vi "Share data.vi"(8 "error in (no error)":errorcluster) -> (0 "error out":errorcluster)   [LabVIEW 2015]
uses:
  shared data (name value unit).ctl
  available share data.ctl
  selected shared data.ctl
  share data command.ctl
panel:
  out "Array 3":i32[](array[numeric])
  out "Array 2":i32[](array[numeric])
  out "Array":dbl[](array[numeric])
  out "Selected Shared Data":T1
  out "Cumulative shared data sizes":i32[](array[numeric])
  out "Selected elements":i32[](array[numeric])
  in  "Tab Control":T2(tab)
  out "My data to share":T3 {"scaled" format="%.2f"}
  in  "Write":bool[](array[boolean])
  in  "My data scrollbar":i32(c297)
  in  "List of available data":i32[](listbox)
  out "Available shared data":T4 {"Shared Data"."scaled" format="%.2f"}
  in  "Data update interval (s)":sgl=5.0 min=5 max=1000 step=5
  in  "Shared Folder":path
  in  "OK":bool
  # "The share data feature enables sharing of sensor, meter, and calculated values between workstations in a laboratory. Data acquired by this instance of ProCoDA can be shared with other ProCoDA applications and shared data from other ProCoDA applications can be accessed here.\n\nSelect a shared folder that can be accessed by all ProCoDA applications that will be sharing data.\nSet the Data update interval based on the rate at which data changes. This controls both the rate at which data is written to file and read from file.\n\nOnce data sharing is configured and initiated by a data source, then it will be visible in the \"Shared data from other instances of ProCoDA\" tab.\n\nAll available data from this computer (sensors and variables) is compiled in an array and the values that are shared are based on the selected indices in the \"My data to share\" tab. Thus if the available data is modified it will shift the array and the shared variable will change. Thus it is recommended that sharing of values be used cautiously if the ProCoDA method is still being edited.\n\nShared data is read from the files based on the name of the variable. If the name of the variable is changed by the data source, then reselect the variable using this dialog box. \n\nSelect the shared data to read by highlighting the row. Multiple rows can be selected by holding the control button down while clicking."
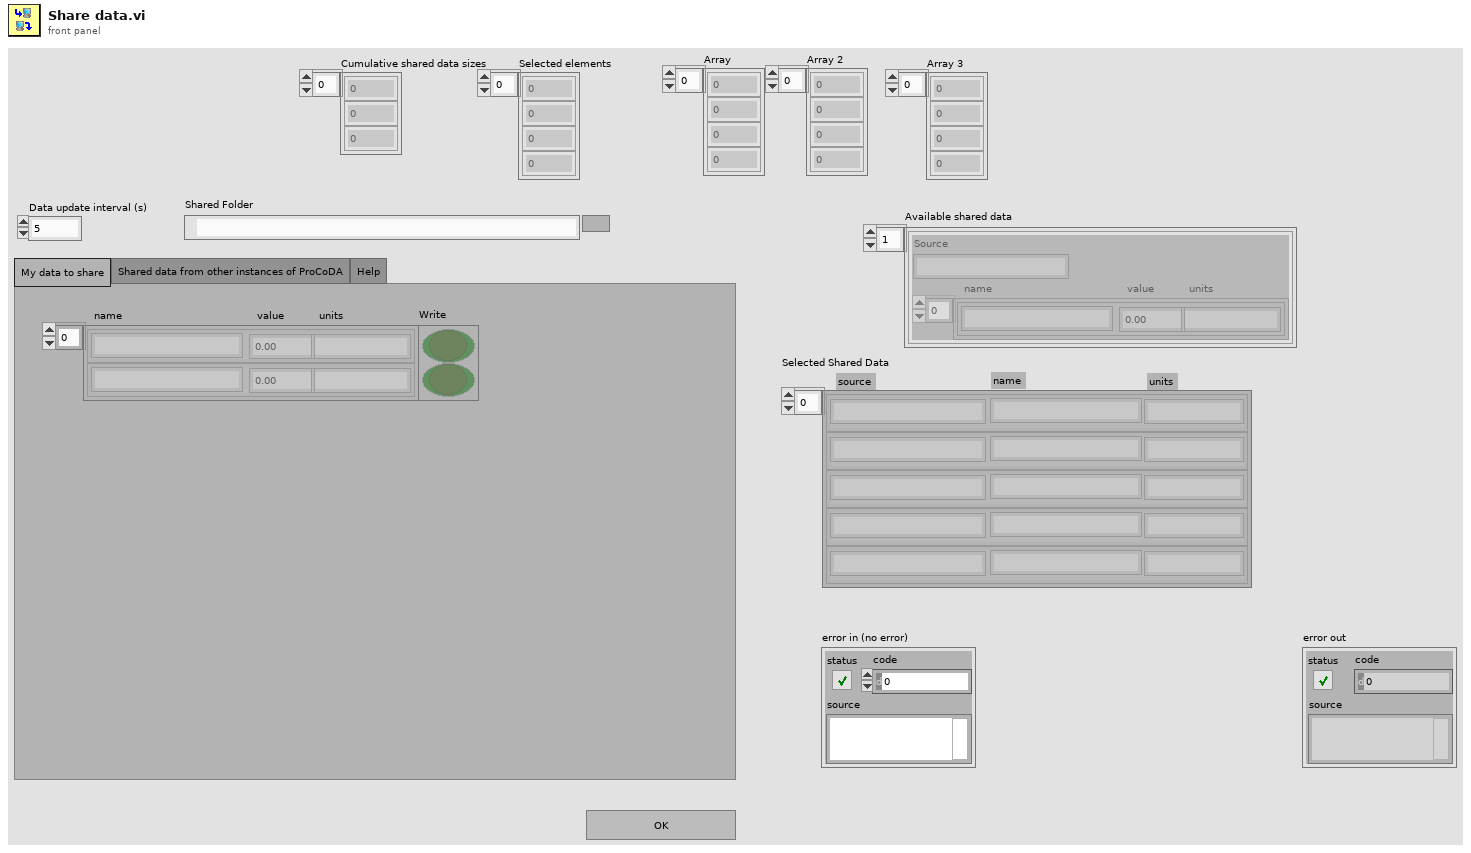
[diagram p1: front panel]
types:
  T1 = typedef "selected shared data.ctl" = cluster{"Source":string, "name":string, "units":string}[]
  T2 = enum32{"My data to share", "Shared data from other instances of ProCoDA", "Help"}
  T3 = typedef "shared data (name value unit).ctl" = cluster{"name":string, "units":string, "scaled":sgl}[]
  T4 = typedef "available share data.ctl" = cluster{"Source":string, "Shared Data":T3}[]
  T5 = typedef "share data command.ctl" = enum16{"Initialize from ini", "Update ini", "Write data", "Read data", "List my data", "List shared data", "Close"}
  T6 = cluster{"Source":string, "name":string, "units":string}
  T7 = cluster{"name":string, "units":string, "scaled":sgl}
  T8 = cluster{"Data update interval (s)":sgl, "Shared Folder":path, "Write":bool[]}
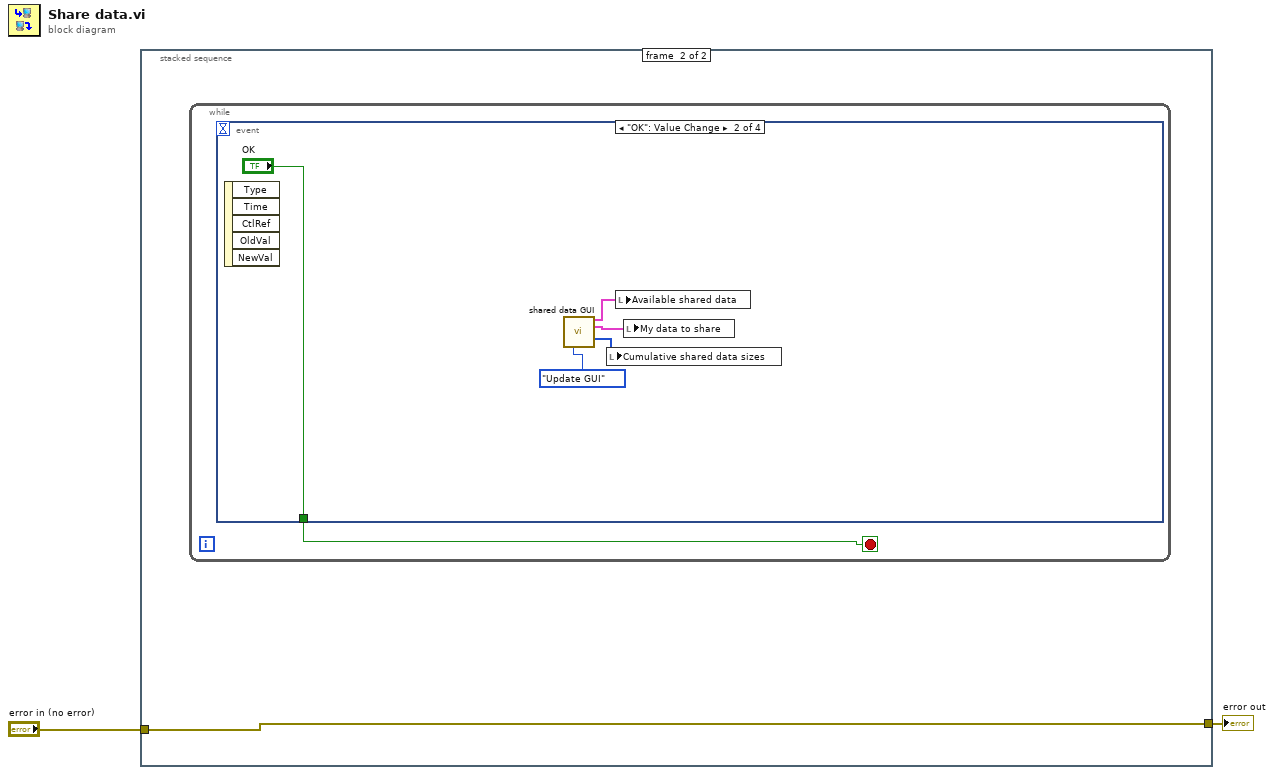
[diagram p0: block diagram]
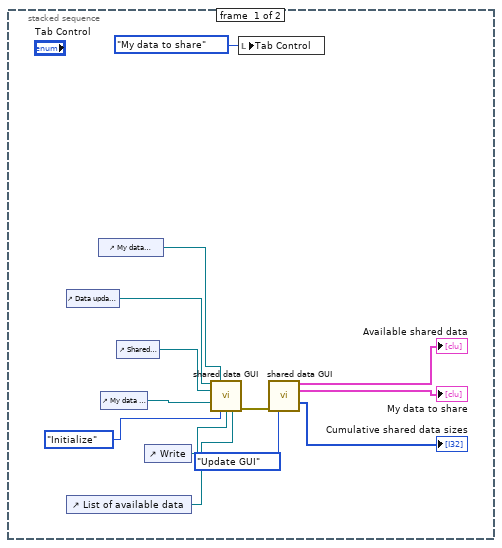
[diagram p2: hidden frame]
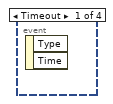
[diagram p3: hidden frame]
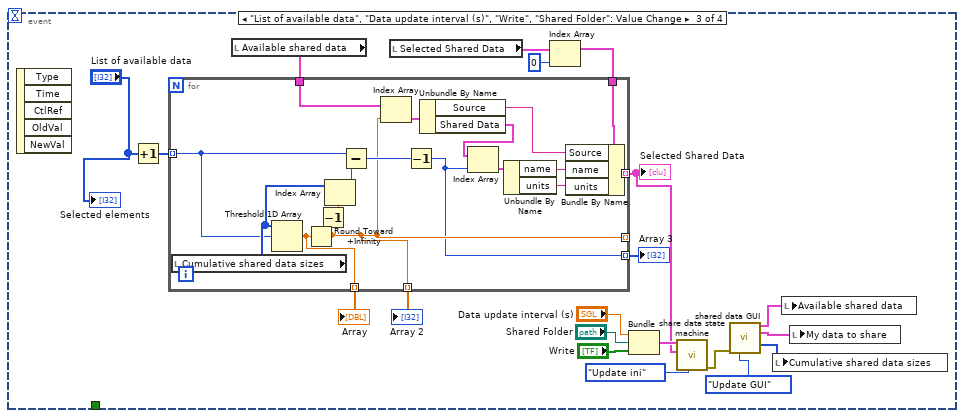
[diagram p4: hidden frame]
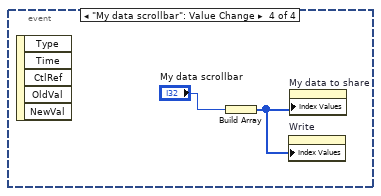
[diagram p5: hidden frame]
diagram:
  n1 = stacked-sequence {
    tunnel: [_ w16] -> w2
    tunnel: "error in (no error)" -> [_ w16]
    frame #0 {
      n2 = control-ref of="Data update interval (s)"() -> (w9:refnum<vi>)
      n3 = control-ref of="List of available data"() -> (w10:refnum<vi>)
      n4 = control-ref of="My data scrollbar"() -> (w14:refnum<vi>)
      n5 = control-ref of="My data to share"() -> (w12:refnum<vi>)
      n6 = control-ref of="Shared Folder"() -> (w13:refnum<vi>)
      n7 = control-ref of="Write"() -> (w11:refnum<vi>)
      n8 = call "shared data GUI.vi"("data update interval"=w9, "Scroll Refnum"=w14, "shared folder"=w13, "My data to share"=w12, "command"=enum16{"Initialize", "Update GUI"}."Initialize", "Write"=w11, "List of available data"=w10) -> ("error out"=w7:errorcluster)  [unwired: 5 in, 3 out]
      n9 = local write "Tab Control"(T2."My data to share" ("Tab Control")) -> ()
      n10 = call "shared data GUI.vi"("error in (no error)"=w7, "command"=enum16{"Initialize", "Update GUI"}."Update GUI") -> ("Available shared data"=→"Available shared data":T4, "My data to share"=→"My data to share":T3, "Cumulative shared data sizes"=→"Cumulative shared data sizes":i32[])  [unwired: 10 in, 1 out]
    }
    frame #1 {
      n11 = while {
        stop <- w17 stop-if-true
        n12 = event shown="[1] \"OK\": Value Change" {
          selector: _ -> [_ _ _ _]
          dyn-events: _ -> [_ _ _ _]
          timeout: _ -> [_ _ _ _]
          tunnel: [_ "OK" _ _] -> w17
          event Timeout {
            n13 = event-data() -> ()  [unwired: 1 in, 2 out]
          }
          event "OK": Value Change {
            n14 = event-data() -> ()  [unwired: 1 in, 5 out]
            n15 = call "shared data GUI.vi"("command"=enum16{"Initialize", "Update GUI"}."Update GUI") -> ("Available shared data"=w18:T4, "My data to share"=w19:T3, "Cumulative shared data sizes"=w20:i32[])  [unwired: 11 in, 1 out]
            n16 = local write "Cumulative shared data sizes"(w20) -> ()
            n17 = local write "Available shared data"(w18) -> ()
            n18 = local write "My data to share"(w19) -> ()
          }
          event "List of available data", "Data update interval (s)", "Write", "Shared Folder": Value Change {
            n19 = event-data() -> ()  [unwired: 1 in, 5 out]
            n20 = Increment(x="List of available data") -> (x+1=w24:i32[])
            n21 = local read "Available shared data"() -> (w42:T4)
            n22 = local read "Selected Shared Data"() -> (w41:T1)
            n23 = Index Array(array=w41, index=0) -> (element=w34:T6)
            n24 = for {
              tunnel: w24 -> [w57] mode=indexing
              tunnel: [w45] -> _ mode=indexing
              tunnel: [w43] -> w23 mode=indexing
              tunnel: w42 -> [w56]
              tunnel: w34 -> [w51]
              tunnel: [w48] -> w32 mode=indexing
              tunnel: [w46] -> w26 mode=indexing
              tunnel: [w45] -> w25 mode=indexing
              n25 = local read "Cumulative shared data sizes"() -> (w59:i32[])
              n26 = Threshold 1D Array(2:w57, 3:w59) -> (0:w46:dbl)  [unwired: 1 in]
              n27 = Round Toward +Infinity(x=w46) -> (ceil(x): smallest int >= x=w45:dbl)
              n28 = Decrement(x=w45) -> (x-1=w44:dbl)
              n29 = Index Array(array=w59, index=w44) -> (element=w58:i32)
              n30 = Subtract(x=w57, y=w58) -> (x-y=w47:i32)
              n31 = Index Array(array=w56, index=w45) -> (element=w55:cluster{"Source":string, "Shared Data":T3})
              n32 = Decrement(x=w47) -> (x-1=w43:i32)
              n33 = Unbundle By Name(w55) -> ("Source"=w49:string, "Shared Data"=w54:T3)
              n34 = Index Array(array=w54, index=w43) -> (element=w53:T7)
              n35 = Unbundle By Name(w53) -> ("name"=w52:string, "units"=w50:string)
              n36 = Bundle By Name(cluster=w51, "Source"=w49, "name"=w52, "units"=w50) -> (w48:T6)
            }
            "Selected Shared Data" <- w32
            "Array" <- w26
            "Array 2" <- w25
            "Array 3" <- w23
            n37 = Bundle("Data update interval (s)"="Data update interval (s)", "Shared Folder"="Shared Folder", "Write"="Write") -> (w37:T8)  [unwired: 1 in]
            n38 = call "share data state machine.vi"("Share data command"=share_data_command."Update ini", "Selected Shared Data"=w32, "Write data cluster in"=w37) -> ("error out"=w27:errorcluster)  [unwired: 2 in, 6 out]
            n39 = call "shared data GUI.vi"("error in (no error)"=w27, "command"=enum16{"Initialize", "Update GUI"}."Update GUI") -> ("Available shared data"=w28:T4, "My data to share"=w29:T3, "Cumulative shared data sizes"=w30:i32[])  [unwired: 10 in, 1 out]
            n40 = local write "Cumulative shared data sizes"(w30) -> ()
            n41 = local write "Available shared data"(w28) -> ()
            n42 = local write "My data to share"(w29) -> ()
            "Selected elements" <- "List of available data"
          }
          event "My data scrollbar": Value Change {
            n43 = event-data() -> ()  [unwired: 1 in, 5 out]
            n44 = Build Array("My data scrollbar") -> (w60:i32[])
            n45 = property on="Write" class="Arr (strict)"("Index Values"=w60) -> ()  [unwired: 2 in, 2 out]
            n46 = property on="My data to share" class="Arr (strict)"("Index Values"=w60) -> ()  [unwired: 2 in, 2 out]
          }
        }
      }
    }
  }
  "error out" <- w2
